vi "Histogram.vi"() -> ()   [LabVIEW 2016]
uses:
  Typedefs/Histogram--slider.ctl
  Typedefs/Histogram--Graph.ctl
  graph_utilities.lvclass/graph_utilities.ctl
  graph_utilities.lvclass
panel:
  in  "lock to bin edges":bool
  out "Histogram":T1
  out "Intensity Graph":dbl[][](graph)
  in  "# std deviations for histogram width":T2=1.4340101522842639 scale=0.0..5.0
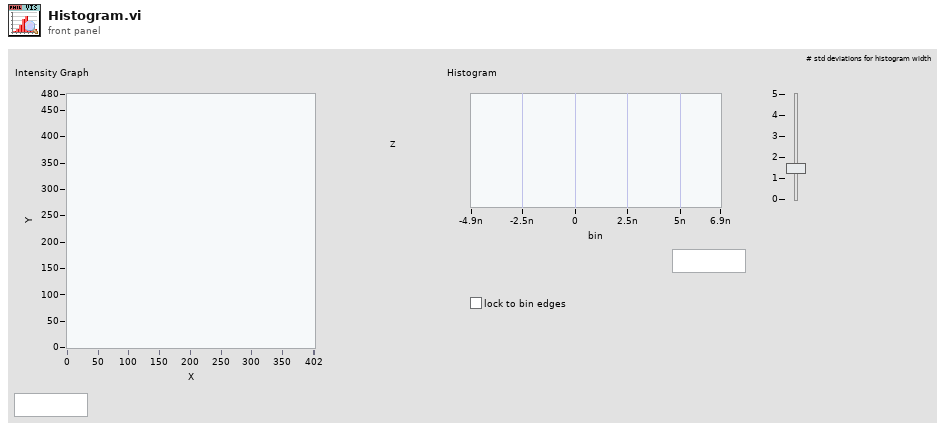
[diagram p1: front panel]
types:
  T1 = typedef "graph_utilities.lvclass/Histogram--Graph.ctl" = cluster{"X":dbl, "Y":dbl}[]
  T2 = typedef "graph_utilities.lvclass/Histogram--slider.ctl" = dbl
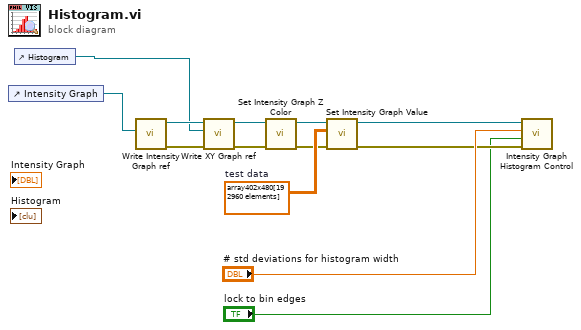
[diagram p0: block diagram]
diagram:
  w12 = dbl[][] array402x480[192960 elements]  # test data
  n1 = control-ref of="Intensity Graph"() -> (w10:refnum<vi>)
  n2 = control-ref of="Histogram"() -> (w1:refnum<vi>)
  n3 = call "Write Intensity Graph ref.vi"("Intensity Graph"=w10) -> ("error out"=w7:errorcluster, "graph_utilities out"=w6:refnum<class "graph_utilities.lvclass">)  [unwired: 9 in]
  n4 = call "Write XY Graph ref.vi"("error in (no error)"=w7, "XY Graph"=w1, "graph_utilities in"=w6) -> ("error out"=w4:errorcluster, "graph_utilities out"=w5:refnum<class "graph_utilities.lvclass">)  [unwired: 7 in]
  n5 = call "Set Intensity Graph Z Color.vi"("error in (no error)"=w4, "graph_utilities in"=w5) -> ("error out"=w11:errorcluster, "graph_utilities out"=w13:refnum<class "graph_utilities.lvclass">)  [unwired: 8 in]
  n6 = call "Set Intensity Graph Value.vi"("error in (no error)"=w11, "Value"=w12, "graph_utilities in"=w13) -> ("error out"=w3:errorcluster, "graph_utilities out"=w9:refnum<class "graph_utilities.lvclass">)  [unwired: 7 in]
  n7 = call "Intensity Graph Histogram Control.vi"("error in (no error)"=w3, "lock to bin edges"="lock to bin edges", "# std deviations for histogram width"="# std deviations for histogram width", "graph_utilities in"=w9) -> ()  [unwired: 4 in, 4 out]
